vi "VI Tree.vi"   [LabVIEW 2020, in "Olympus IX BX Series.lvlib"]
doc: "This is the instrument driver for the OLYMPUS IX2, BX2A Microscope.\n\nThe VI Tree displays all the user-callable VIs of the instrument driver in an organized table."
uses:
  Olympus IX BX Series.lvlib
panel:
  # "© 2005 National Instruments.  ALL RIGHTS RESERVED."
  # "SEE DIAGRAM\nFOR VI TREE."
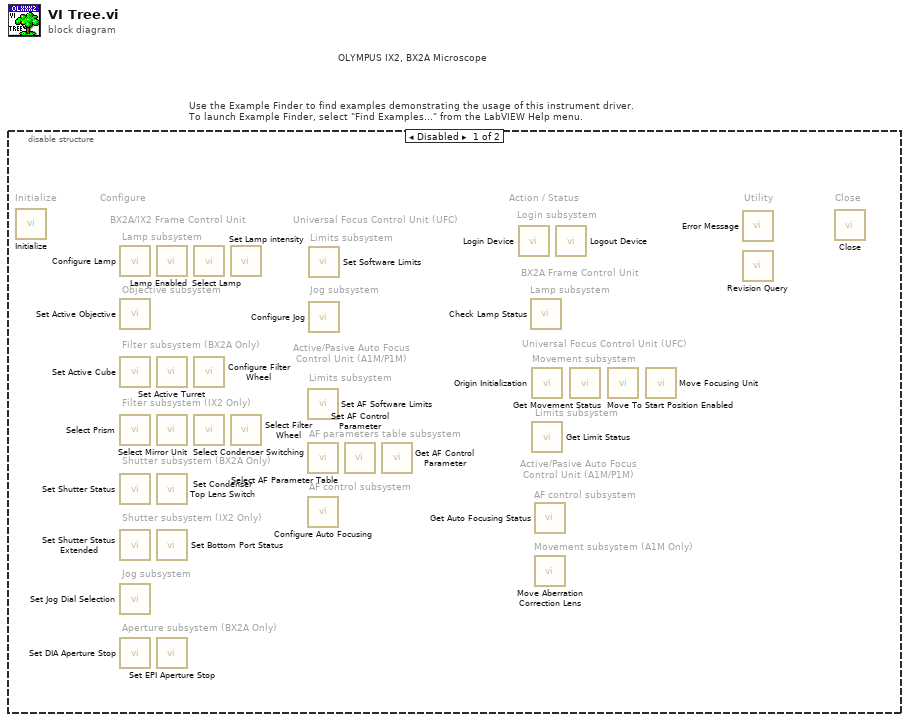
[diagram p0: block diagram]
diagram:
  # "Use the Example Finder to find examples demonstrating the usage of this instrument driver.\nTo launch Example Finder, select \"Find Examples...\" from the LabVIEW Help menu."
  # "OLYMPUS IX2, BX2A Microscope"
  n1 = disable-structure shown="Disabled" {
    frame Disabled {
      # "Active/Pasive Auto Focus\n Control Unit (A1M/P1M)"
      # "AF control subsystem"
      # "Limits subsystem"
      # "Movement subsystem"
      # "Universal Focus Control Unit (UFC)"
      # "BX2A Frame Control Unit"
      # "Lamp subsystem"
      # "Close"
      # "Utility"
      # "Action / Status"
      # "Configure"
      # "Initialize"
      # "Shutter subsystem (IX2 Only)"
      # "Filter subsystem (IX2 Only)"
      # "Jog subsystem"
      # "Movement subsystem (A1M Only)"
      # "AF control subsystem"
      # "AF parameters table subsystem"
      # "Limits subsystem"
      # "Active/Pasive Auto Focus\n Control Unit (A1M/P1M)"
      # "Jog subsystem"
      # "Limits subsystem"
      # "Universal Focus Control Unit (UFC)"
      # "Aperture subsystem (BX2A Only)"
      # "Shutter subsystem (BX2A Only)"
      # "Filter subsystem (BX2A Only)"
      # "Objective subsystem"
      # "Lamp subsystem"
      # "Login subsystem"
      # "BX2A/IX2 Frame Control Unit"
      n2 = call "Initialize.vi"() -> ()  [unwired: 14 in, 2 out]
      n3 = call "Configure Lamp.vi"() -> ()  [unwired: 14 in, 2 out]
      n4 = call "Set Active Objective.vi"() -> ()  [unwired: 10 in, 2 out]
      n5 = call "Set Active Cube.vi"() -> ()  [unwired: 10 in, 2 out]
      n6 = call "Select Prism.vi"() -> ()  [unwired: 10 in, 2 out]
      n7 = call "Set Shutter Status.vi"() -> ()  [unwired: 10 in, 2 out]
      n8 = call "Set Shutter Status Extended.vi"() -> ()  [unwired: 14 in, 2 out]
      n9 = call "Set Jog Dial Selection.vi"() -> ()  [unwired: 10 in, 2 out]
      n10 = call "Set DIA Aperture Stop.vi"() -> ()  [unwired: 10 in, 2 out]
      n11 = call "Lamp Enabled.vi"() -> ()  [unwired: 10 in, 2 out]
      n12 = call "Set Active Turret.vi"() -> ()  [unwired: 10 in, 2 out]
      n13 = call "Select Mirror Unit.vi"() -> ()  [unwired: 10 in, 2 out]
      n14 = call "Set Condenser Top Lens Switch.vi"() -> ()  [unwired: 10 in, 2 out]
      n15 = call "Set Bottom Port Status.vi"() -> ()  [unwired: 10 in, 2 out]
      n16 = call "Set EPI Aperture Stop.vi"() -> ()  [unwired: 10 in, 2 out]
      n17 = call "Select Lamp.vi"() -> ()  [unwired: 10 in, 2 out]
      n18 = call "Configure Filter Wheel.vi"() -> ()  [unwired: 14 in, 2 out]
      n19 = call "Select Condenser Switching.vi"() -> ()  [unwired: 10 in, 2 out]
      n20 = call "Set Lamp intensity.vi"() -> ()  [unwired: 10 in, 2 out]
      n21 = call "Select Filter Wheel.vi"() -> ()  [unwired: 10 in, 2 out]
      n22 = call "Set AF Software Limits.vi"() -> ()  [unwired: 14 in, 2 out]
      n23 = call "Select AF Parameter Table.vi"() -> ()  [unwired: 10 in, 2 out]
      n24 = call "Configure Auto Focusing.vi"() -> ()  [unwired: 14 in, 2 out]
      n25 = call "Set Software Limits.vi"() -> ()  [unwired: 14 in, 2 out]
      n26 = call "Configure Jog.vi"() -> ()  [unwired: 14 in, 2 out]
      n27 = call "Set AF Control Parameter.vi"() -> ()  [unwired: 14 in, 2 out]
      n28 = call "Get AF Control Parameter.vi"() -> ()  [unwired: 9 in, 3 out]
      n29 = call "Login Device.vi"() -> ()  [unwired: 10 in, 2 out]
      n30 = call "Check Lamp Status.vi"() -> ()  [unwired: 9 in, 3 out]
      n31 = call "Origin Initialization.vi"() -> ()  [unwired: 10 in, 2 out]
      n32 = call "Get Limit Status.vi"() -> ()  [unwired: 9 in, 3 out]
      n33 = call "Get Auto Focusing Status.vi"() -> ()  [unwired: 13 in, 3 out]
      n34 = call "Move Aberration Correction Lens.vi"() -> ()  [unwired: 14 in, 2 out]
      n35 = call "Logout Device.vi"() -> ()  [unwired: 10 in, 2 out]
      n36 = call "Get Movement Status.vi"() -> ()  [unwired: 9 in, 3 out]
      n37 = call "Move To Start Position Enabled.vi"() -> ()  [unwired: 10 in, 2 out]
      n38 = call "Move Focusing Unit.vi"() -> ()  [unwired: 14 in, 2 out]
      n39 = call "Error Message.vi"() -> ()  [unwired: 11 in, 5 out]
      n40 = call "Revision Query.vi"() -> ()  [unwired: 12 in, 4 out]
      n41 = call "Close.vi"() -> ()  [unwired: 15 in, 1 out]
    }
    frame Enabled {
    }
  }
